vi "hmp4000 Configure Output State Channel Only.vi"(8 "error in (no error)":errorcluster, 9 "Output State (Off)":bool, 11 "VISA resource name":refnum<visa-resource-name>) -> (0 "error out":errorcluster, 3 "VISA resource name out":refnum<visa-resource-name>)   [LabVIEW 2022 SP3]
doc: "Turns the channel output ON or OFF. Compared to hmp4000 Configure Output State.vi, it doesn't change the General output switch settings.\n\nAttribute:\nHMP4000_ATTR_OUTPUT_SELECT\n\nRemote-control command:\nOUTPut:SELect"
uses:
  Instance           1 38Saved   hmp4000 Configure Output State .vi
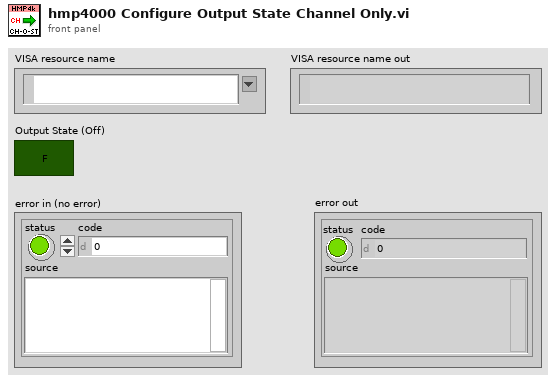
[diagram p1: front panel]
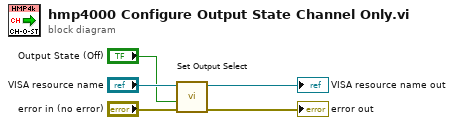
[diagram p0: block diagram]
diagram:
  n1 = call "Set Output Select"("error in (no error)"="error in (no error)", "Output Select (OFF)"="Output State (Off)", "instrument handle"="VISA resource name") -> ("error out"=→"error out":errorcluster, "instrument handle out"=→"VISA resource name out":refnum<visa-resource-name>)  [unwired: 7 in]
